vi "L5K Extract for MCLB.vi"(8 "error in":errorcluster, 11 "L5K Information":T1) -> (0 "error out":errorcluster, 3 "Tag Info for MCLB":string[][](array[string]))   [LabVIEW 2023, in "Ethernet IP Custom Device Custom Device.lvlib"]
uses:
  Ethernet IP Custom Device Custom Device.lvlib
  L5K Internal Data.ctl
  L5K Tag.ctl
  L5K Data Types.ctl
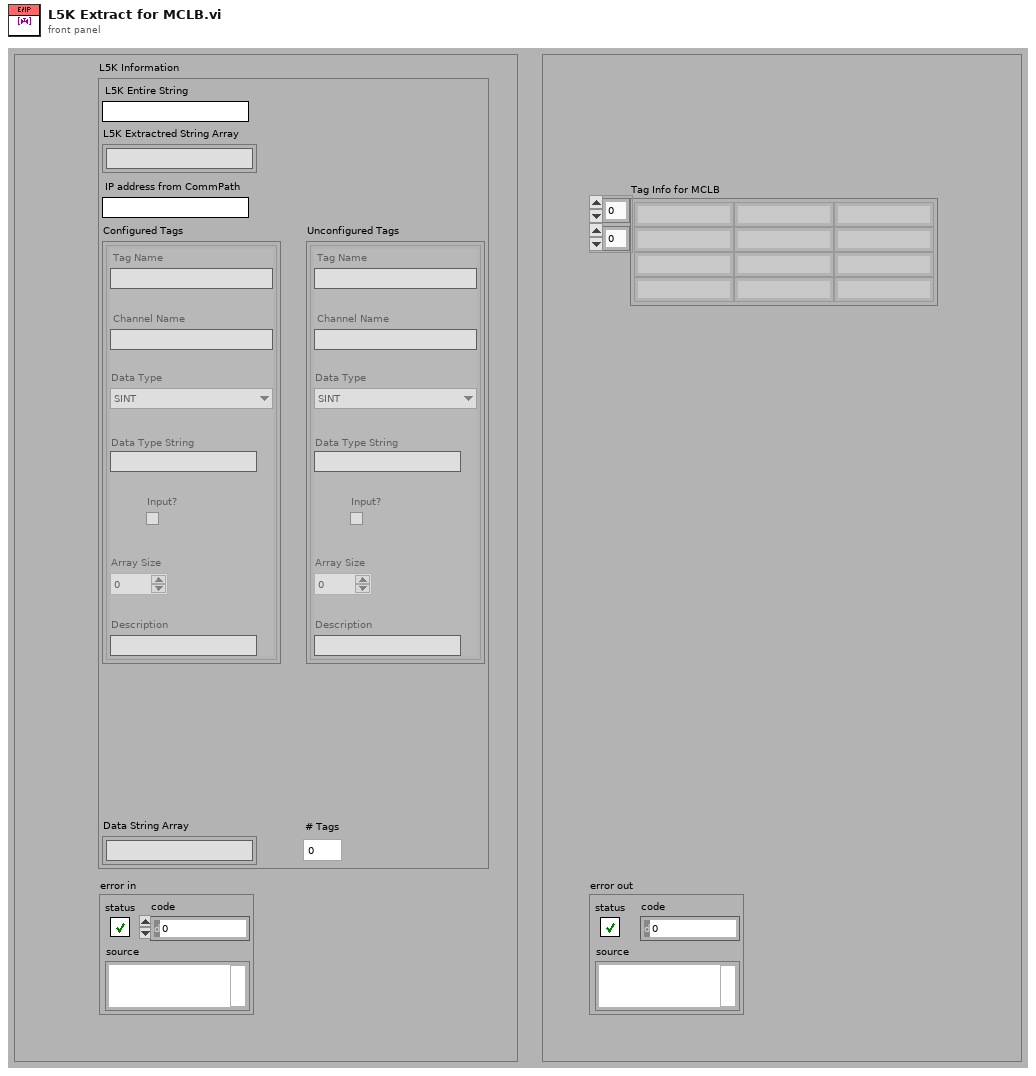
[diagram p1: front panel]
types:
  T1 = typedef "Ethernet IP Custom Device Custom Device.lvlib/L5K Internal Data.ctl" = cluster{"L5K Entire String":string, "L5K Extractred String Array":string[], "IP address from CommPath":string, "Configured Tags":T2[], "Data String Array":string[], "Unconfigured Tags":T2[], "# Tags":i32}
  T2 = typedef "Ethernet IP Custom Device Custom Device.lvlib/L5K Tag.ctl" = cluster{"Tag Name":string, "Data Type":T3, "Data Type String":string, "Array Size":i32, "Description":string, "Input?":bool, "Channel Name":string}
  T3 = typedef "Ethernet IP Custom Device Custom Device.lvlib/L5K Data Types.ctl" = enum16{"SINT", "INT", "DINT", "REAL", "BOOL"}
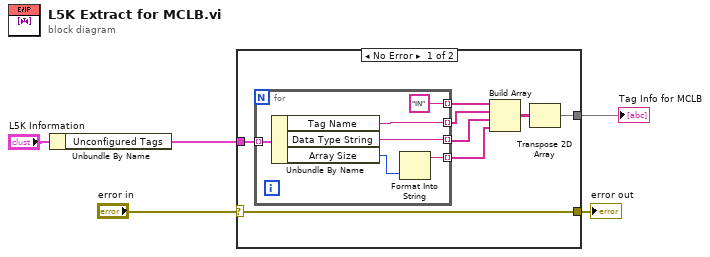
[diagram p0: block diagram]
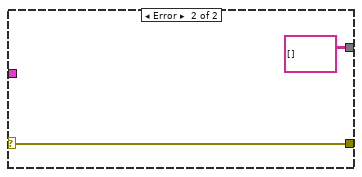
[diagram p2: hidden frame]
diagram:
  n1 = Unbundle By Name("L5K Information") -> ("Unconfigured Tags"=w1:T2[])
  n2 = case shown="No Error" "error in" {
    selector: "error in" -> [w9 w20]
    tunnel: [w10 string[][] []] -> w3
    tunnel: [w9 w20] -> w5
    tunnel: w1 -> [w8 _]
    frame No Error {
      n3 = for {
        tunnel: [w19] -> w7 mode=indexing
        tunnel: [w18] -> w6 mode=indexing
        tunnel: [w17] -> w12 mode=indexing
        tunnel: ["IN"] -> w13 mode=indexing
        tunnel: w8 -> [w15] mode=indexing
        n4 = Unbundle By Name(w15) -> ("Tag Name"=w19:string, "Data Type String"=w18:string, "Array Size"=w14:i32)
        n5 = Format Into String(w14) -> (resulting string=w17:string)  [unwired: 3 in, 1 out]
      }
      n6 = Build Array(w13, w7, w6, w12) -> (w11:string[][])
      n7 = Transpose 2D Array(2D array=w11) -> (transposed array=w10:string[][])
    }
    frame Error {
    }
  }
  "Tag Info for MCLB" <- w3
  "error out" <- w5
